vi "Get Node Info.vi"(8 "error in (no error)":errorcluster, 10 "Active Build Configuration":string, 11 "Caraya Item in":refnum<class "Caraya Item.lvclass">) -> (0 "error out":errorcluster, 1 "Child Nodes":refnum<class "Node.lvclass">[](array[class]), 2 "Label":string)   [LabVIEW 2019, in "Caraya Library.lvlib" / "Caraya Item.lvclass"]
uses:
  Caraya Item.lvclass
  libs/Solution.lvlibp/Solution/Tree Entry/Node.lvclass
  Caraya Item.lvclass/Caraya Item.ctl
  Caraya Library.lvlib
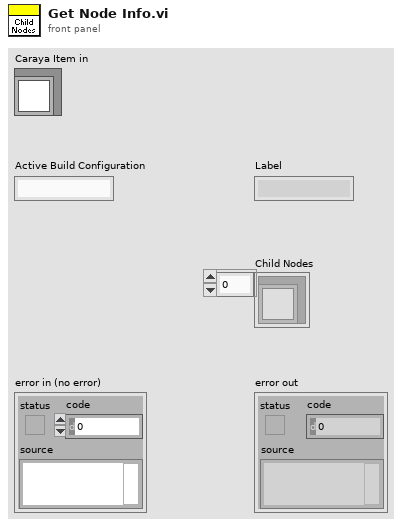
[diagram p1: front panel]
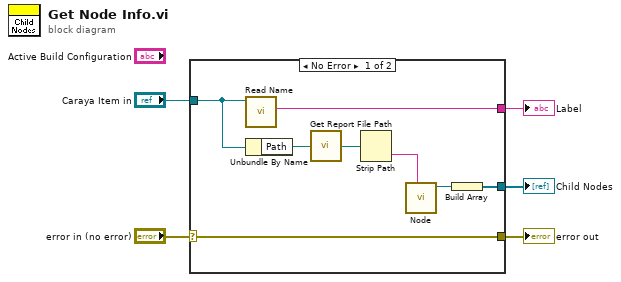
[diagram p0: block diagram]
diagram:
  n1 = case shown="No Error" "error in (no error)" {
    selector: "error in (no error)" -> [w6 w14]
    tunnel: [w13 _] -> w5
    tunnel: "Caraya Item in" -> [w11 _]
    tunnel: [w8 _] -> w3
    tunnel: [w6 w14] -> w1
    frame No Error {
      n2 = call-dynamic "Read Name.vi"("Caraya Item in"=w11) -> ("Name"=w13:string)  [unwired: 10 in]
      n3 = Unbundle By Name(w11) -> ("Path"=w10:path)
      n4 = call "Get Report File Path.vi"("Path"=w10) -> ("Report File"=w12:path)  [unwired: 1 in]
      n5 = Strip Path(path=w12) -> (name=w7:string)  [unwired: 1 out]
      n6 = call "Node.vi"("Name"=w7) -> ("Tree Entry out"=w9:refnum<class "Node.lvclass">)  [unwired: 10 in]
      n7 = Build Array(w9) -> (w8:refnum<class "Node.lvclass">[])
    }
    frame Error {
    }
  }
  "error out" <- w1
  "Child Nodes" <- w3
  "Label" <- w5
